vi "4Pi Sample Focus Control.vi"(7 "Calling VI Ref":refnum<vi>) -> ()   [LabVIEW 2016]
uses:
  4Pi Sample Focus Controls/Focus Control.ctl
  4Pi Sample Focus Controls/XY Navigation.ctl
  <vilib>/Utility/miscctls.llb/LVPointTypeDef.ctl
  Hardware Configuration/Hardware Configuration Controls/Device Function.ctl
  Hardware Configuration/Hardware Configuration Controls/Device Type.ctl
  Device Library/Stages/Stages Controls/Stage Actions.ctl
  Device Library/Shutters/Shutter Controls/Shutter Actions.ctl
panel:
  in  "Toggle Shutters":bool
  in  "Lower Shutter":bool
  in  "Upper Shutter":bool
  in  "Quit":bool
  in  "Lower Objective XY":T1 {"XY Step Size (µm)" format="%#_4g"; "Y Position (µm)" format="%#_4g"; "X Position (µm)" format="%#_4g"}
  in  "Upper Objective Focus":T2 {"Step Size (µm)" format="%#_4g"}
  in  "Z Stage Focus":T2 {"Step Size (µm)" format="%#_4g"}
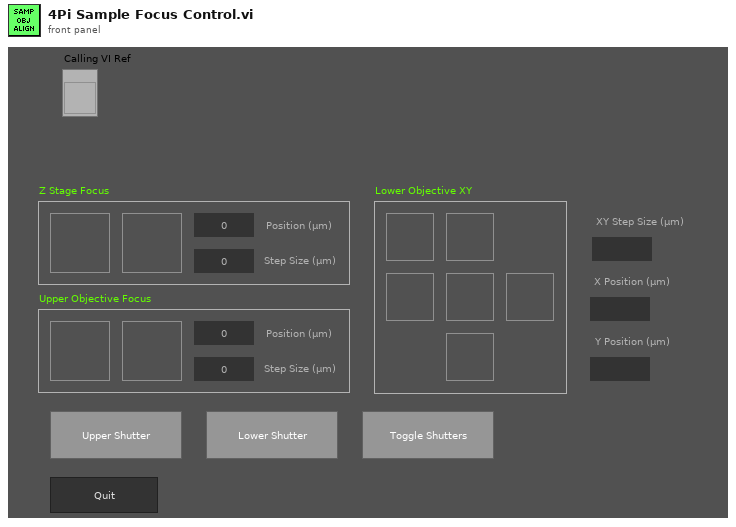
[diagram p1: front panel]
types:
  T1 = typedef "XY Navigation.ctl" = cluster{"Up":bool, "Halt":bool, "Down":bool, "Left":bool, "Right":bool, "Home":bool, "X Position (µm)":dbl, "Y Position (µm)":dbl, "XY Step Size (µm)":dbl}
  T2 = typedef "Focus Control.ctl" = cluster{"Z Up":bool, "Z Down":bool, "Position (µm)":dbl, "Step Size (µm)":dbl}
  T3 = enum16{"Always On", "Always Off", "Off While Running"}
  T4 = typedef "LVPointTypeDef.ctl" = cluster{"Horizontal":i16, "Vertical":i16}
  T5 = typedef "Device Function.ctl" = enum16{"Primary", "Secondary", "Overview", "Wide Field Drift Correction", "642 nm Excitation", "560 nm Excitation", "546 nm Excitation", "488 nm Excitation", "405 nm Excitation", "Objective Drift Correction", "Objective XY", "Objective Z", "Sample XY", "Sample Coarse Z", "Sample Z", "4Pi Lower", "4Pi Upper", "Adj Cavity"}
  T6 = typedef "Device Type.ctl" = enum16{"AOTF", "Camera", "Deformable Mirror", "Laser", "Shutter", "Stage"}
  T7 = typedef "Shutter Actions.ctl" = enum16{"Open", "Close", "Toggle", "Status", "Quit"}
  T8 = typedef "Stage Actions.ctl" = enum16{"Get Position", "MVR", "MOVE", "HALT", "ONTARGET", "ERROR", "REFERENCE", "INIT", "VELOCITY", "STATUS", "EXIT", "HOME", "ZEROPOS", "NANOPOS", "ANALOG", "QUIT"}
  T9 = cluster{"Z Up":bool, "Z Down":bool, "Position (µm)":bool, "Step Size (µm)":bool}
  T10 = cluster{"Up":bool, "Halt":bool, "Down":bool, "Left":bool, "Right":bool, "Home":bool, "X Position (µm)":bool, "Y Position (µm)":bool, "XY Step Size (µm)":bool}
  T11 = typedef "LVRectTypeDef.ctl" = cluster{"Left":i16, "Top":i16, "Right":i16, "Bottom":i16}
  T12 = typedef "LVBoundsTypeDef.ctl" = cluster{"Width":u32, "Height":u32}
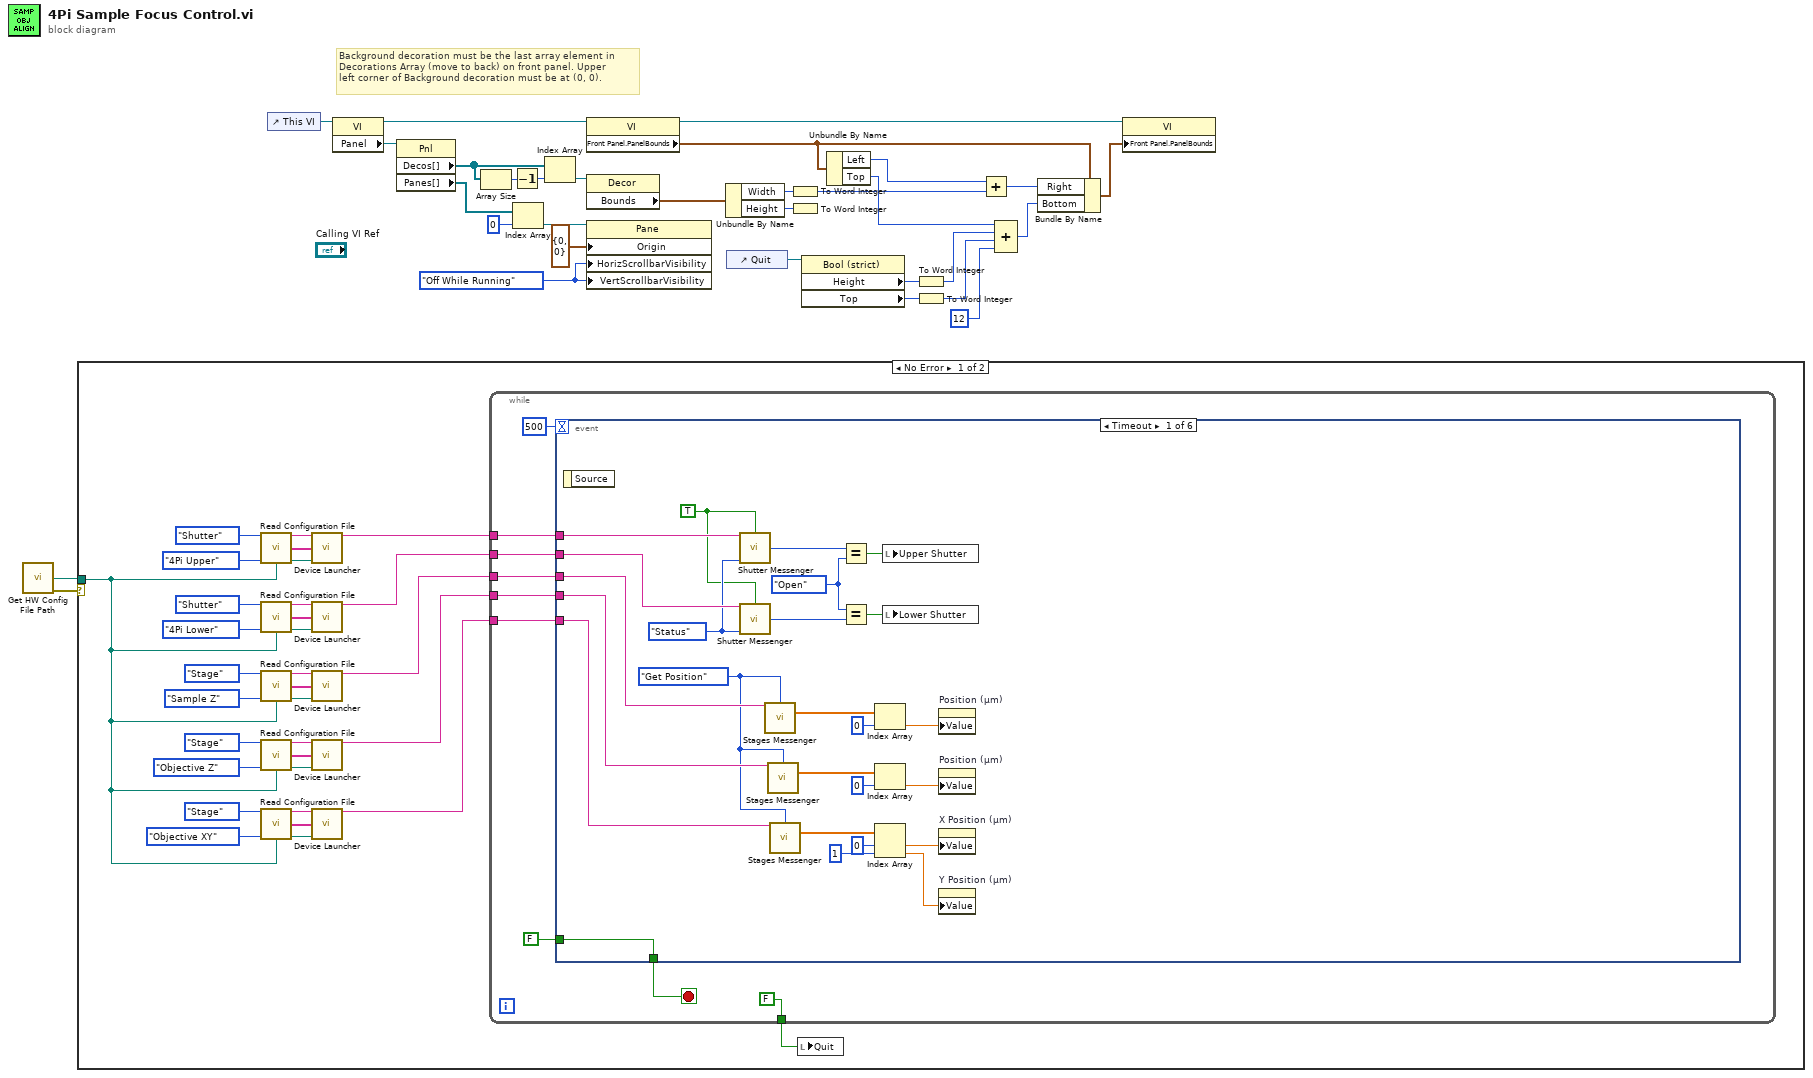
[diagram p0: block diagram]
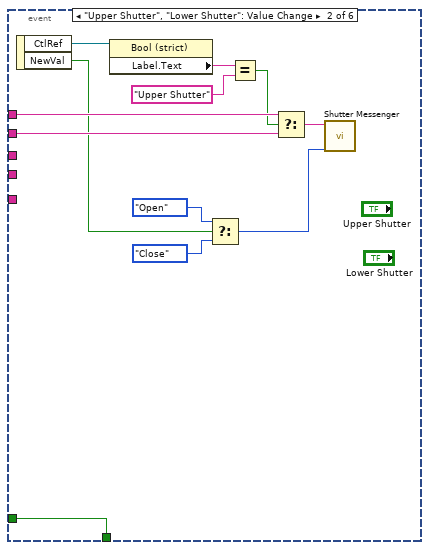
[diagram p2: hidden frame]
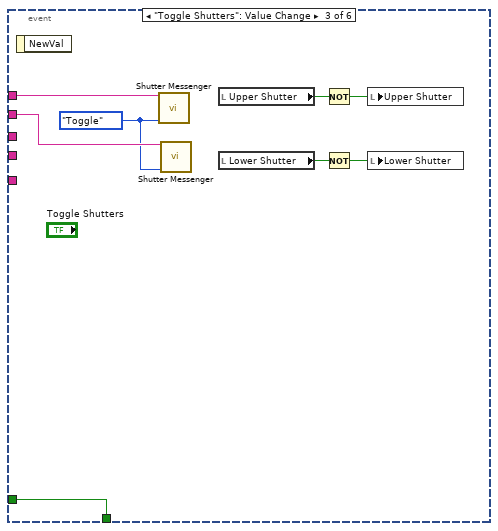
[diagram p3: hidden frame]
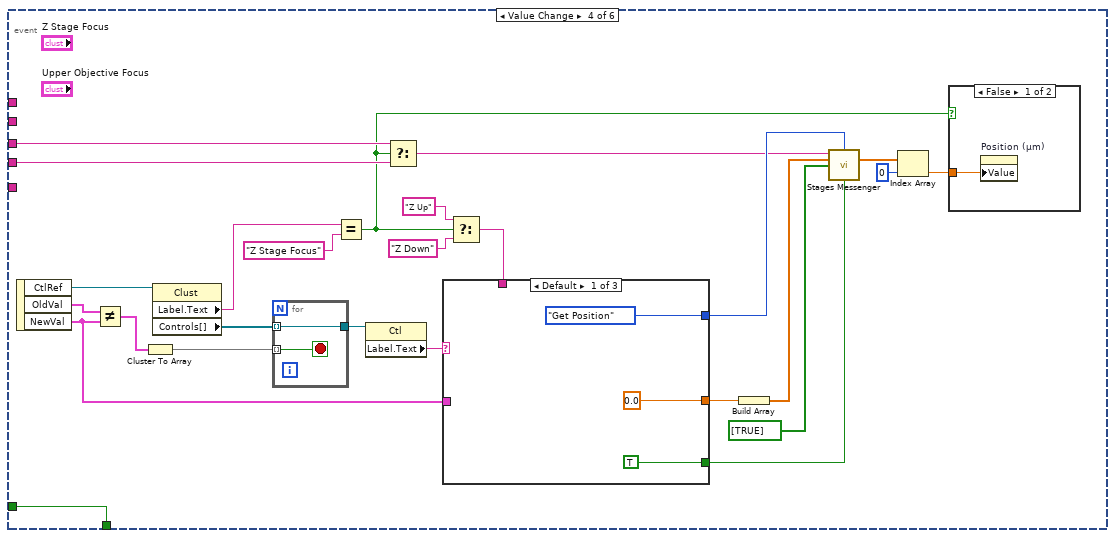
[diagram p4: hidden frame]
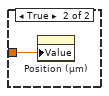
[diagram p5: hidden frame]
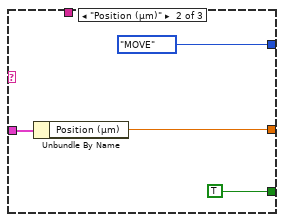
[diagram p6: hidden frame]
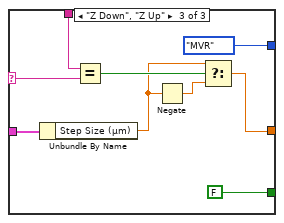
[diagram p7: hidden frame]
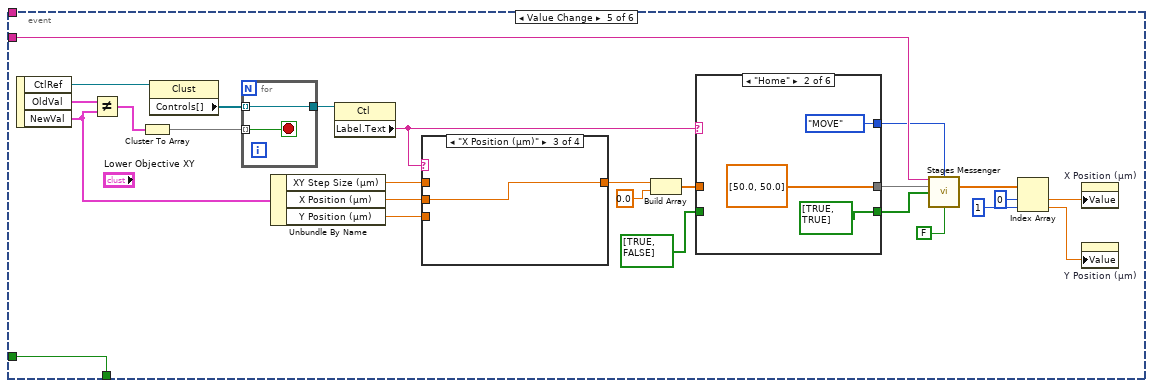
[diagram p8: hidden frame]
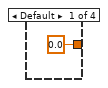
[diagram p9: hidden frame]
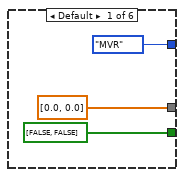
[diagram p12: hidden frame]
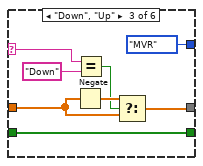
[diagram p13: hidden frame]
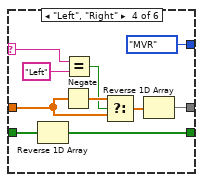
[diagram p14: hidden frame]
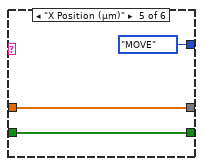
[diagram p15: hidden frame]
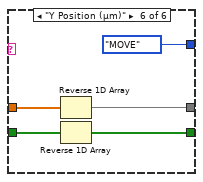
[diagram p16: hidden frame]
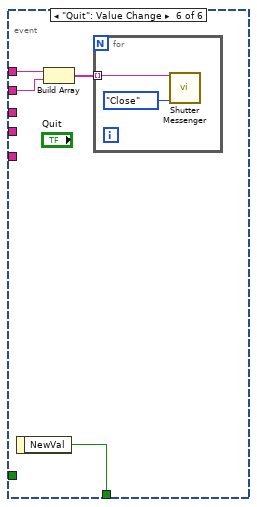
[diagram p17: hidden frame]
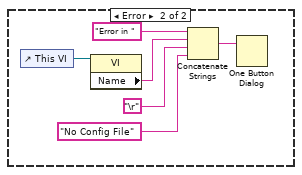
[diagram p18: hidden frame]
diagram:
  w14 = T3."Off While Running" ("Vertical Scrollbar Visibility")
  # "Background decoration must be the last array element in\nDecorations Array (move to back) on front panel. Upper\nleft corner of Background decoration must be at (0, 0)."
  n1 = call "Get HW Config File Path.vi"() -> ("File Path"=w2:path, "Error"=w1:errorcluster)  [unwired: 14 in]
  n2 = case shown="No Error" w1 {
    tunnel: w2 -> [w36 _]
    frame No Error {
      n3 = call "Read Configuration File.vi"("Device Type"=Device_Type."Shutter", "Device Function"=Device_Function."4Pi Upper", "Config File Path"=w36) -> ("Unique Notifier Name"=w62:string, "Device Ports/IDs/Channels"=w61:string[], "Device Engine Path"=w60:path)  [unwired: 9 in, 1 out]
      n4 = call "Read Configuration File.vi"("Device Type"=Device_Type."Shutter", "Device Function"=Device_Function."4Pi Lower", "Config File Path"=w36) -> ("Unique Notifier Name"=w53:string, "Device Ports/IDs/Channels"=w54:string[], "Device Engine Path"=w55:path)  [unwired: 9 in, 1 out]
      n5 = call "Read Configuration File.vi"("Device Type"=Device_Type."Stage", "Device Function"=Device_Function."Sample Z", "Config File Path"=w36) -> ("Unique Notifier Name"=w41:string, "Device Ports/IDs/Channels"=w40:string[], "Device Engine Path"=w39:path)  [unwired: 9 in, 1 out]
      n6 = call "Read Configuration File.vi"("Device Type"=Device_Type."Stage", "Device Function"=Device_Function."Objective Z", "Config File Path"=w36) -> ("Unique Notifier Name"=w42:string, "Device Ports/IDs/Channels"=w43:string[], "Device Engine Path"=w44:path)  [unwired: 9 in, 1 out]
      n7 = call "Read Configuration File.vi"("Device Type"=Device_Type."Stage", "Device Function"=Device_Function."Objective XY", "Config File Path"=w36) -> ("Unique Notifier Name"=w51:string, "Device Ports/IDs/Channels"=w50:string[], "Device Engine Path"=w49:path)  [unwired: 9 in, 1 out]
      n8 = call "Device Launcher.vi"("Notifier Name"=w62, "Device Ports/IDs/Channels"=w61, "Device Engine Path"=w60) -> ("Notifier Name"=w52:string)  [unwired: 11 in, 1 out]
      n9 = call "Device Launcher.vi"("Notifier Name"=w53, "Device Ports/IDs/Channels"=w54, "Device Engine Path"=w55) -> ("Notifier Name"=w63:string)  [unwired: 11 in, 1 out]
      n10 = call "Device Launcher.vi"("Notifier Name"=w41, "Device Ports/IDs/Channels"=w40, "Device Engine Path"=w39) -> ("Notifier Name"=w35:string)  [unwired: 11 in, 1 out]
      n11 = call "Device Launcher.vi"("Notifier Name"=w42, "Device Ports/IDs/Channels"=w43, "Device Engine Path"=w44) -> ("Notifier Name"=w34:string)  [unwired: 11 in, 1 out]
      n12 = call "Device Launcher.vi"("Notifier Name"=w51, "Device Ports/IDs/Channels"=w50, "Device Engine Path"=w49) -> ("Notifier Name"=w33:string)  [unwired: 11 in, 1 out]
      n13 = while {
        tunnel: w52 -> [w71]
        tunnel: w63 -> [w70]
        tunnel: w35 -> [w67]
        tunnel: w34 -> [w66]
        tunnel: w33 -> [w65]
        tunnel: [FALSE] -> w32
        stop <- w68 stop-if-true
        n14 = event shown="[0] Timeout" {
          selector: _ -> [_ _ _ _ _ _]
          dyn-events: _ -> [_ _ _ _ _ _]
          timeout: 500 -> [_ _ _ _ _ _]
          tunnel: w71 -> [w81 w108 w116 _ _ w230]
          tunnel: w70 -> [w80 w107 w115 _ _ w229]
          tunnel: FALSE -> [w97 w105 w117 w143 w189 _]
          tunnel: [w97 w105 w117 w143 w189 w231] -> w68
          tunnel: w67 -> [w96 _ _ w127 _ _]
          tunnel: w66 -> [w95 _ _ w126 _ _]
          tunnel: w65 -> [w94 _ _ _ w177 _]
          event Timeout {
            w75 = Shutter_Actions."Open" ("y")
            w78 = TRUE ("Quick Status")
            w79 = Shutter_Actions."Status" ("Action")
            w93 = Stage_Actions."Get Position" ("Actions")
            n15 = event-data() -> ()  [unwired: 1 in, 1 out]
            n16 = call "Shutter Messenger.vi"("Notifier Name"=w81, "Quick Status"=w78, "Action"=w79) -> ("Shutter Status"=w77:T7)  [unwired: 11 in, 1 out]
            n17 = call "Shutter Messenger.vi"("Notifier Name"=w80, "Quick Status"=w78, "Action"=w79) -> ("Shutter Status"=w76:T7)  [unwired: 11 in, 1 out]
            n18 = call "Stages Messenger.vi"("Stage Notifier Name"=w96, "Actions"=w93) -> ("Positions"=w92:dbl[])  [unwired: 10 in, 3 out]
            n19 = call "Stages Messenger.vi"("Stage Notifier Name"=w95, "Actions"=w93) -> ("Positions"=w88:dbl[])  [unwired: 10 in, 3 out]
            n20 = call "Stages Messenger.vi"("Stage Notifier Name"=w94, "Actions"=w93) -> ("Positions"=w87:dbl[])  [unwired: 10 in, 3 out]
            n21 = Equal?(x=w77, y=w75) -> (x = y?=w74:bool)
            n22 = Equal?(x=w75, y=w76) -> (x = y?=w73:bool)
            n23 = Index Array(array=w92, index=0) -> (element=w82:dbl)
            n24 = Index Array(array=w88, index=0) -> (element=w83:dbl)
            n25 = Index Array(array=w87, index #1=0 ("index"), index #2=1 ("index")) -> (element #1=w85:dbl, element #2=w84:dbl)
            n26 = local write "Upper Shutter"(w74) -> ()
            n27 = local write "Lower Shutter"(w73) -> ()
            n28 = property on="Position (µm)" class="DigNum (strict)"("Value"=w82) -> ()  [unwired: 2 in, 2 out]
            n29 = property on="Position (µm)" class="DigNum (strict)"("Value"=w83) -> ()  [unwired: 2 in, 2 out]
            n30 = property on="X Position (µm)" class="DigNum (strict)"("Value"=w85) -> ()  [unwired: 2 in, 2 out]
            n31 = property on="Y Position (µm)" class="DigNum (strict)"("Value"=w84) -> ()  [unwired: 2 in, 2 out]
          }
          event "Upper Shutter", "Lower Shutter": Value Change {
            n32 = event-data() -> ("CtlRef"=w109:refnum<vi>, "NewVal"=w106:bool)  [unwired: 1 in]
            n33 = property class="Bool (strict)"(reference=w109) -> ("Label.Text"=w104:string)  [unwired: 1 in, 2 out]
            n34 = Select(t=Shutter_Actions."Open" ("Action"), s=w106, f=Shutter_Actions."Close" ("Action")) -> (s? t:f=w98:T7)
            n35 = Equal?(x=w104, y="Upper Shutter") -> (x = y?=w102:bool)
            n36 = Select(t=w108, s=w102, f=w107) -> (s? t:f=w101:string)
            n37 = call "Shutter Messenger.vi"("Notifier Name"=w101, "Action"=w98) -> ()  [unwired: 12 in, 2 out]
          }
          event "Toggle Shutters": Value Change {
            w114 = Shutter_Actions."Toggle" ("Action")
            n38 = event-data() -> ()  [unwired: 1 in, 1 out]
            n39 = call "Shutter Messenger.vi"("Notifier Name"=w116, "Action"=w114) -> ()  [unwired: 12 in, 2 out]
            n40 = call "Shutter Messenger.vi"("Notifier Name"=w115, "Action"=w114) -> ()  [unwired: 12 in, 2 out]
            n41 = local read "Upper Shutter"() -> (w113:bool)
            n42 = local read "Lower Shutter"() -> (w112:bool)
            n43 = Not(x=w113) -> (.not. x?=w111:bool)
            n44 = Not(x=w112) -> (.not. x?=w110:bool)
            n45 = local write "Upper Shutter"(w111) -> ()
            n46 = local write "Lower Shutter"(w110) -> ()
          }
          event Value Change {
            n47 = event-data() -> ("CtlRef"=w142:refnum<vi>, "OldVal"=w141:T2, "NewVal"=w135:T2)  [unwired: 1 in]
            n48 = Not Equal?(x=w141, y=w135) -> (x != y?=w139:T9)
            n49 = Cluster To Array(cluster=w139) -> (array=w138:bool[])
            n50 = property class="Clust"(reference=w142) -> ("Label.Text"=w129:string, "Controls[]"=w140:refnum<vi>[])  [unwired: 1 in, 2 out]
            n51 = for {
              tunnel: w140 -> [w162] mode=indexing
              tunnel: w138 -> [w163] mode=indexing
              tunnel: [w162] -> w137
              stop <- w163 stop-if-true
            }
            n52 = Equal?(x=w129, y="Z Stage Focus") -> (x = y?=w119:bool)
            n53 = property class="Ctl"(reference=w137) -> ("Label.Text"=w136:string)  [unwired: 1 in, 2 out]
            n54 = Select(t=w127, s=w119, f=w126) -> (s? t:f=w125:string)
            n55 = Select(t="Z Up", s=w119, f="Z Down" ("y")) -> (s? t:f=w122:string)
            n56 = case shown="Default" w136 {
              selector: w136 -> [_ _ w154]
              tunnel: w135 -> [_ w151 w161]
              tunnel: [Stage_Actions."Get Position" ("Actions") Stage_Actions."MOVE" ("Actions") Stage_Actions."MVR" ("Actions")] -> w131
              tunnel: [0.0 ("Step Size (µm)") w150 w156] -> w134
              tunnel: [TRUE TRUE FALSE] -> w130
              tunnel: w122 -> [_ _ w153]
              frame Default {
              }
              frame "Position (µm)" {
                n57 = Unbundle By Name(w151) -> ("Position (µm)"=w150:dbl)
              }
              frame "Z Down", "Z Up" {
                n58 = Unbundle By Name(w161) -> ("Step Size (µm)"=w159:dbl)
                n59 = Equal?(x=w153, y=w154) -> (x = y?=w160:bool)
                n60 = Negate(x=w159) -> (-x=w158:dbl)
                n61 = Select(t=w159, s=w160, f=w158) -> (s? t:f=w156:dbl)
              }
            }
            n62 = Build Array(w134) -> (w133:dbl[])
            n63 = call "Stages Messenger.vi"("Stage Notifier Name"=w125, "Actions"=w131, "Setpoint"=w133, "Axis"=bool[] [TRUE], "Exit While Busy?"=w130) -> ("Positions"=w121:dbl[])  [unwired: 7 in, 3 out]
            n64 = Index Array(array=w121, index=0) -> (element=w118:dbl)
            n65 = case shown="False" w119 {
              tunnel: w118 -> [w144 w145]
              frame False {
                n66 = property on="Position (µm)" class="DigNum (strict)"("Value"=w144) -> ()  [unwired: 2 in, 2 out]
              }
              frame True {
                n67 = property on="Position (µm)" class="DigNum (strict)"("Value"=w145) -> ()  [unwired: 2 in, 2 out]
              }
            }
          }
          event Value Change {
            n68 = event-data() -> ("CtlRef"=w185:refnum<vi>, "OldVal"=w184:T1, "NewVal"=w176:T1)  [unwired: 1 in]
            n69 = Not Equal?(x=w184, y=w176) -> (x != y?=w188:T10)
            n70 = Cluster To Array(cluster=w188) -> (array=w187:bool[])
            n71 = property class="Clust"(reference=w185) -> ("Controls[]"=w183:refnum<vi>[])  [unwired: 1 in, 2 out]
            n72 = for {
              tunnel: w183 -> [w226] mode=indexing
              tunnel: w187 -> [w227] mode=indexing
              tunnel: [w226] -> w186
              stop <- w227 stop-if-true
            }
            n73 = Unbundle By Name(w176) -> ("XY Step Size (µm)"=w173:dbl, "X Position (µm)"=w172:dbl, "Y Position (µm)"=w171:dbl)
            n74 = property class="Ctl"(reference=w186) -> ("Label.Text"=w174:string)  [unwired: 1 in, 2 out]
            n75 = case shown="\"X Position (µm)\"" w174 {
              tunnel: w173 -> [_ w191 _ _]
              tunnel: w172 -> [_ _ w192 _]
              tunnel: w171 -> [_ _ _ w193]
              tunnel: [0.0 ("Y Position (µm)") w191 w192 w193] -> w170
              frame Default {
              }
              frame "Down", "Left", "Right", "Up" {
              }
              frame "X Position (µm)" {
              }
              frame "Y Position (µm)" {
              }
            }
            n76 = Build Array(w170, 0.0 ("element")) -> (w181:dbl[])
            n77 = case shown="\"Home\"" w174 {
              selector: w174 -> [_ _ w207 w214 _ _]
              tunnel: w181 -> [_ _ w204 w213 w219 w225]
              tunnel: bool[] [TRUE, FALSE] -> [_ _ w201 w211 w218 w224]
              tunnel: [dbl[] [0.0, 0.0] dbl[] [50.0, 50.0] w203 w210 w219 w223] -> w179
              tunnel: [bool[] [FALSE, FALSE] bool[] [TRUE, TRUE] w201 w209 w218 w222] -> w178
              tunnel: [Stage_Actions."MVR" ("Actions") Stage_Actions."MOVE" ("Actions") Stage_Actions."MVR" ("Actions") Stage_Actions."MVR" ("Actions") Stage_Actions."MOVE" ("Actions") Stage_Actions."MOVE" ("Actions")] -> w175
              frame Default {
              }
              frame "Home" {
              }
              frame "Down", "Up" {
                n78 = Negate(x=w204) -> (-x=w205:dbl[])
                n79 = Equal?(x=w207, y="Down") -> (x = y?=w202:bool)
                n80 = Select(t=w205, s=w202, f=w204) -> (s? t:f=w203:dbl[])
              }
              frame "Left", "Right" {
                n81 = Reverse 1D Array(array=w211) -> (reversed array=w209:bool[])
                n82 = Negate(x=w213) -> (-x=w216:dbl[])
                n83 = Equal?(x=w214, y="Left") -> (x = y?=w215:bool)
                n84 = Select(t=w216, s=w215, f=w213) -> (s? t:f=w212:dbl[])
                n85 = Reverse 1D Array(array=w212) -> (reversed array=w210:dbl[])
              }
              frame "X Position (µm)" {
              }
              frame "Y Position (µm)" {
                n86 = Reverse 1D Array(array=w225) -> (reversed array=w223:dbl[])
                n87 = Reverse 1D Array(array=w224) -> (reversed array=w222:bool[])
              }
            }
            n88 = call "Stages Messenger.vi"("Stage Notifier Name"=w177, "Actions"=w175, "Setpoint"=w179, "Axis"=w178, "Exit While Busy?"=FALSE) -> ("Positions"=w164:dbl[])  [unwired: 7 in, 3 out]
            n89 = Index Array(array=w164, index #1=0 ("index"), index #2=1 ("index")) -> (element #1=w166:dbl, element #2=w165:dbl)
            n90 = property on="X Position (µm)" class="DigNum (strict)"("Value"=w166) -> ()  [unwired: 2 in, 2 out]
            n91 = property on="Y Position (µm)" class="DigNum (strict)"("Value"=w165) -> ()  [unwired: 2 in, 2 out]
          }
          event "Quit": Value Change {
            n92 = event-data() -> ("NewVal"=w231:bool)  [unwired: 1 in]
            n93 = Build Array(w230, w229) -> (w228:string[])
            n94 = for {
              tunnel: w228 -> [w233] mode=indexing
              n95 = call "Shutter Messenger.vi"("Notifier Name"=w233, "Action"=Shutter_Actions."Close") -> ()  [unwired: 12 in, 2 out]
            }
          }
        }
      }
      n96 = local write "Quit"(w32) -> ()
    }
    frame Error {
      n97 = control-ref of="This VI"() -> (w239:refnum<vi>)
      n98 = property class="VI"(reference=w239) -> ("Name"=w237:string)  [unwired: 1 in, 2 out]
      n99 = Concatenate Strings("Error in ", w237, "\r", "No Config File") -> (w234:string)
      n100 = One Button Dialog(message=w234) -> ()  [unwired: 1 in, 1 out]
    }
  }
  n101 = control-ref of="This VI"() -> (w7:refnum<vi>)
  n102 = property class="VI"(reference=w7) -> (reference out=w15:refnum<vi>, "Panel"=w8:refnum<vi>)  [unwired: 1 in, 1 out]
  n103 = property class="Pnl"(reference=w8) -> ("Decos[]"=w6:refnum<vi>[], "Panes[]"=w11:refnum<vi>[])  [unwired: 1 in, 2 out]
  n104 = Array Size(array=w6) -> (size(s)=w4:i32)
  n105 = Decrement(x=w4) -> (x-1=w5:i32)
  n106 = Index Array(array=w11, index=0) -> (element=w10:refnum<vi>)
  n107 = Index Array(array=w6, index=w5) -> (element=w13:refnum<vi>)
  n108 = property class="VI"(reference=w15) -> (reference out=w17:refnum<vi>, "Front Panel.PanelBounds"=w18:T11)  [unwired: 1 in, 1 out]
  n109 = property class="Decor"(reference=w13) -> ("Bounds"=w16:T12)  [unwired: 1 in, 2 out]
  n110 = property class="Pane"(reference=w10, "Origin"=T4 {"Horizontal"=0, "Vertical"=0}, "HorizScrollbarVisibility"=w14, "VertScrollbarVisibility"=w14) -> ()  [unwired: 1 in, 2 out]
  n111 = Unbundle By Name(w16) -> ("Width"=w21:u32, "Height"=w24:u32)
  n112 = control-ref of="Quit"() -> (w3:refnum<vi>)
  n113 = To Word Integer(number=w21) -> (16bit integer=w23:i16)
  n114 = To Word Integer(number=w24) -> ()  [unwired: 1 out]
  n115 = property class="Bool (strict)"(reference=w3) -> ("Height"=w26:u32, "Top"=w27:i32)  [unwired: 1 in, 2 out]
  n116 = Unbundle By Name(w18) -> ("Left"=w20:i16, "Top"=w31:i16)
  n117 = To Word Integer(number=w26) -> (16bit integer=w29:i16)
  n118 = To Word Integer(number=w27) -> (16bit integer=w30:i16)
  n119 = Add(x=w20, y=w23) -> (x+y=w22:i16)
  n120 = Compound Arithmetic op=ADD(w31, w29, w30, i16 12 ("y")) -> (w25:i16)
  n121 = Bundle By Name(cluster=w18, "Right"=w22, "Bottom"=w25) -> (w19:T11)
  n122 = property class="VI"(reference=w17, "Front Panel.PanelBounds"=w19) -> ()  [unwired: 1 in, 2 out]
